vi "Configure Active Meter.vi"(0 "VISA resource name":refnum<visa-resource-name>, 5 "Active Meter (0:Frequency)":u16(ring) items=["Frequency", "Peak Current", "Power", "Current", "Power Factor"], 11 "error in (no error)":errorcluster) -> (4 "VISA resource name out":refnum<visa-resource-name>, 15 "error out":errorcluster)   [LabVIEW 2014, in "eec 6700.lvlib"]
doc: "Sets <B>active meter</B> on the display of the power source instrument."
uses:
  <instrlib>/eec 6700/eec 6700.lvlib
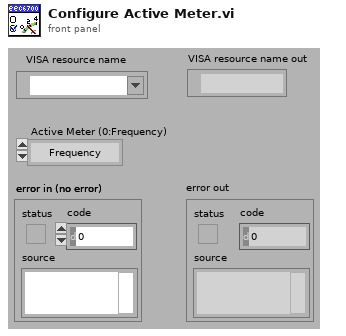
[diagram p1: front panel]
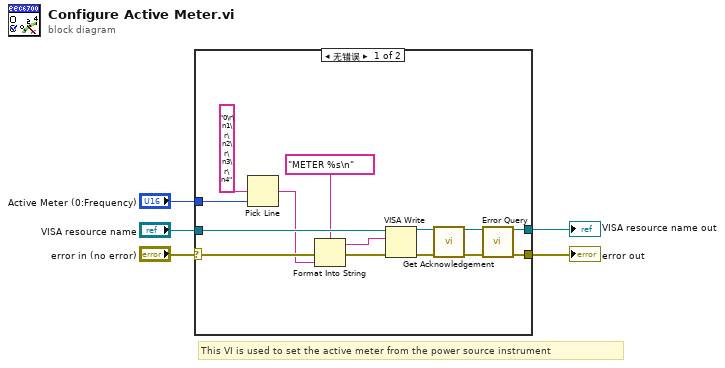
[diagram p0: block diagram]
diagram:
  # "This VI is used to set the active meter from the power source instrument"
  n1 = case shown="无错误" "error in (no error)" {
    selector: "error in (no error)" -> [w12 w20]
    tunnel: "VISA resource name" -> [w19 w21]
    tunnel: "Active Meter (0:Frequency)" -> [w17 _]
    tunnel: [w16 w21] -> w3
    tunnel: [w15 w20] -> w2
    frame No Error {
      n2 = Pick Line(multi-line string="0\r\n1\r\n2\r\n3\r\n4" ("options"), line index=w17) -> (output string=w10:string)  [unwired: 1 in]
      n3 = Format Into String(format string="METER %s\n" ("command"), error in=w12, w10) -> (resulting string=w13:string, error out=w11:errorcluster)  [unwired: 1 in]
      n4 = VISA Write(VISA resource name=w19, write buffer=w13, error in (no error)=w11) -> (VISA resource name out=w8:refnum<visa-resource-name>, error out=w7:errorcluster)  [unwired: 1 out]
      n5 = call <instrlib>:"Get Acknowledgement.vi"("VISA resource name"=w8, "error in (no error)"=w7) -> ("VISA resource name out"=w9:refnum<visa-resource-name>, "error out"=w6:errorcluster)  [unwired: 12 in]
      n6 = call <instrlib>:"Error Query.vi"("VISA resource name"=w9, "error in (no error)"=w6) -> ("VISA resource name out"=w16:refnum<visa-resource-name>, "error out"=w15:errorcluster)  [unwired: 10 in, 2 out]
    }
    frame Error {
    }
  }
  "VISA resource name out" <- w3
  "error out" <- w2
